vi "NetworkTable get.vi"   [LabVIEW 2014]
uses:
  <vilib>/Rock Robotics/Network Tables/SD Read Number.vi
  <vilib>/Rock Robotics/Network Tables/SD Read Boolean.vi
  <vilib>/Rock Robotics/Network Tables/SD Write Number.vi
  <vilib>/Rock Robotics/Network Tables/SD Read String.vi
  Robot Values.vi
  <vilib>/Rock Robotics/Network Tables/SD Write String.vi
types:
  T1 = cluster{"Lift Encoder Height Right (cm)":dbl, "Lift Encoder Height Left (cm)":dbl, "Right Prox":bool, "Left Prox":bool, "Gyro Angle":dbl, "Gyro anglar rate":dbl, "Gyro Reset":bool, "Drive encoder Dash reset":bool}
  T2 = cluster{"DriveMode":enum16{"Tank", "Arcade"}, "Is Logitech":bool}
  T3 = cluster{"Lift Position":i32, "Lift Speed Override":dbl, "OverrideTele?":bool, "OverrideDash":bool}
  T4 = cluster{"Tracking Tote?":bool, "ToteRightSpeed":dbl, "ToteLeftSpeed":dbl, "Drive Encoder reset":bool, "Right Wheel \n(Cm)":dbl, "Left Wheel \n(Cm)":dbl}
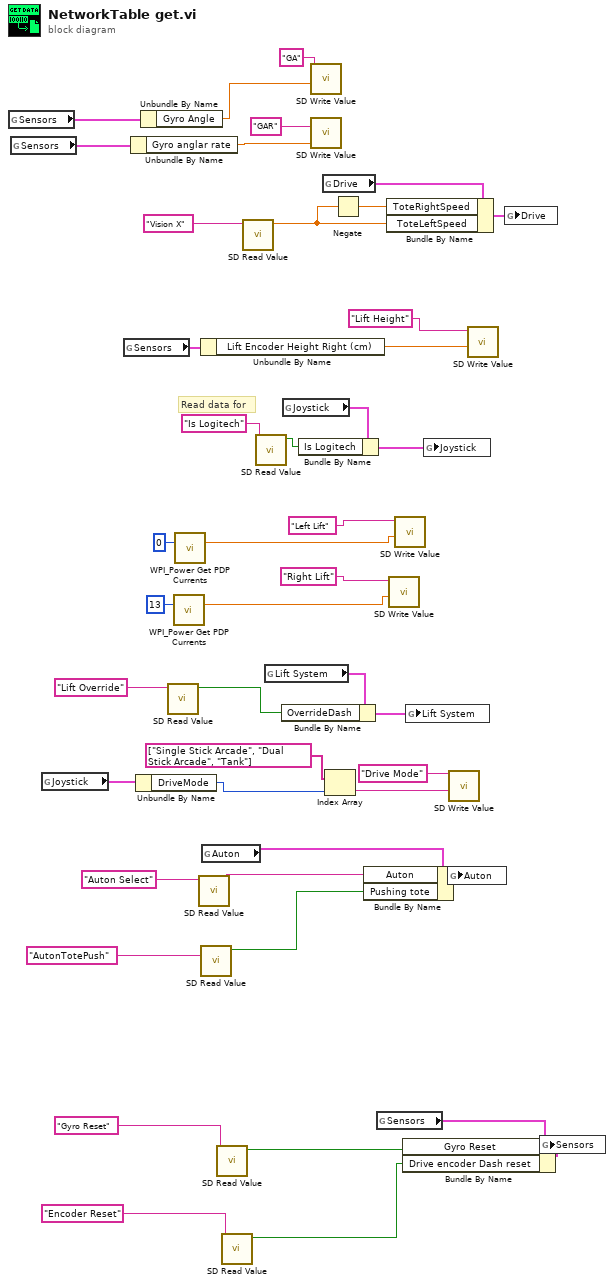
[diagram p0: block diagram]
diagram:
  # "Read data for"
  n1 = global read "Robot Values.vi" "Sensors"() -> (w23:T1)
  n2 = global read "Robot Values.vi" "Sensors"() -> (w22:T1)
  n3 = global read "Robot Values.vi" "Joystick"() -> (w17:T2)
  n4 = global read "Robot Values.vi" "Sensors"() -> (w40:T1)
  n5 = Unbundle By Name(w22) -> ("Gyro anglar rate"=w20:dbl)
  n6 = Unbundle By Name(w17) -> ("DriveMode"=w16:enum16{"Tank", "Arcade"})
  n7 = Unbundle By Name(w23) -> ("Gyro Angle"=w21:dbl)
  n8 = call-poly <vilib>:"SD Read Value.vi"("Name"="Lift Override") -> ("Boolean"=w31:bool)  [unwired: 8 in, 2 out]
  n9 = call <vilib>:"WPI_Power Get PDP Currents.vi"("PDP Channel"=13) -> ("current (A)"=w28:dbl)  [unwired: 12 in, 2 out]
  n10 = call <vilib>:"WPI_Power Get PDP Currents.vi"("PDP Channel"=0) -> ("current (A)"=w26:dbl)  [unwired: 12 in, 2 out]
  n11 = call-poly <vilib>:"SD Read Value.vi"("Name"="Auton Select") -> ("String"=w10:string)  [unwired: 8 in, 2 out]
  n12 = Unbundle By Name(w40) -> ("Lift Encoder Height Right (cm)"=w24:dbl)
  n13 = call-poly <vilib>:"SD Read Value.vi"("Name"="AutonTotePush") -> ("Boolean"=w2:bool)  [unwired: 8 in, 2 out]
  n14 = global read "Robot Values.vi" "Auton"() -> (w11:cluster{"Auton":string, "Pushing tote":bool})
  n15 = call-poly <vilib>:"SD Read Value.vi"("Name"="Gyro Reset") -> ("Boolean"=w6:bool)  [unwired: 8 in, 2 out]
  n16 = call-poly <vilib>:"SD Read Value.vi"("Name"="Encoder Reset") -> ("Boolean"=w3:bool)  [unwired: 8 in, 2 out]
  n17 = call-poly <vilib>:"SD Read Value.vi"("Name"="Vision X") -> ("Numeric"=w41:dbl)  [unwired: 8 in, 2 out]
  n18 = call-poly <vilib>:"SD Read Value.vi"("Name"="Is Logitech") -> ("Boolean"=w37:bool)  [unwired: 8 in, 2 out]
  n19 = global read "Robot Values.vi" "Lift System"() -> (w33:T3)
  n20 = Bundle By Name(cluster=w33, "OverrideDash"=w31) -> (w32:T3)
  n21 = global read "Robot Values.vi" "Joystick"() -> (w38:T2)
  n22 = Bundle By Name(cluster=w38, "Is Logitech"=w37) -> (w36:T2)
  n23 = call-poly <vilib>:"SD Write Value.vi"("Numeric"=w21, "Name"="GA") -> ()  [unwired: 8 in, 2 out]
  n24 = call-poly <vilib>:"SD Write Value.vi"("Numeric"=w20, "Name"="GAR") -> ()  [unwired: 8 in, 2 out]
  n25 = global read "Robot Values.vi" "Drive"() -> (w43:T4)
  n26 = Index Array(array=string[] ["Single Stick Arcade", "Dual Stick Arcade", "Tank"], index=w16) -> (element=w14:string)
  n27 = Negate(x=w41) -> (-x=w42:dbl)
  n28 = Bundle By Name(cluster=w11, "Auton"=w10, "Pushing tote"=w2) -> (w9:cluster{"Auton":string, "Pushing tote":bool})
  n29 = global read "Robot Values.vi" "Sensors"() -> (w8:T1)
  n30 = Bundle By Name(cluster=w43, "ToteRightSpeed"=w42, "ToteLeftSpeed"=w41) -> (w44:T4)
  n31 = call-poly <vilib>:"SD Write Value.vi"("Numeric"=w28, "Name"="Right Lift") -> ()  [unwired: 8 in, 2 out]
  n32 = call-poly <vilib>:"SD Write Value.vi"("Numeric"=w26, "Name"="Left Lift") -> ()  [unwired: 8 in, 2 out]
  n33 = Bundle By Name(cluster=w8, "Gyro Reset"=w6, "Drive encoder Dash reset"=w3) -> (w7:T1)
  n34 = global write "Robot Values.vi" "Lift System"(w32) -> ()
  n35 = global write "Robot Values.vi" "Joystick"(w36) -> ()
  n36 = global write "Robot Values.vi" "Auton"(w9) -> ()
  n37 = call-poly <vilib>:"SD Write Value.vi"("String"=w14, "Name"="Drive Mode") -> ()  [unwired: 8 in, 2 out]
  n38 = call-poly <vilib>:"SD Write Value.vi"("Numeric"=w24, "Name"="Lift Height") -> ()  [unwired: 8 in, 2 out]
  n39 = global write "Robot Values.vi" "Drive"(w44) -> ()
  n40 = global write "Robot Values.vi" "Sensors"(w7) -> ()
